vi "Default.vi"(8 "error in (no error)":errorcluster, 11 "CallEXEStep in":refnum<class "CallEXEStep.lvclass">) -> (0 "error out":errorcluster, 3 "CallEXEStep out":refnum<class "CallEXEStep.lvclass">)   [LabVIEW 2015, in "CallEXEStep.lvclass"]
uses:
  CallEXEStep.lvclass
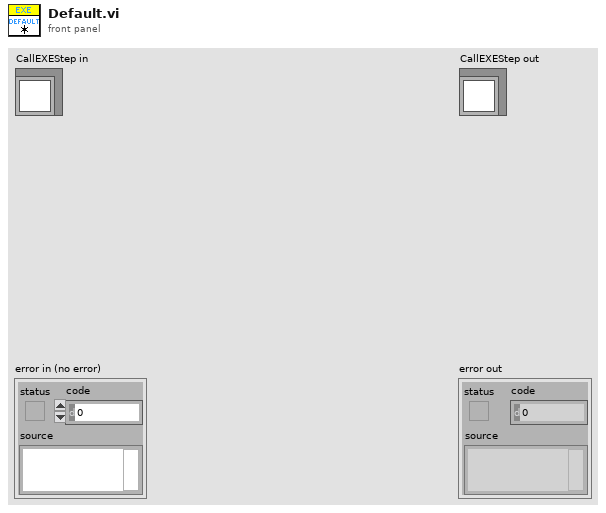
[diagram p1: front panel]
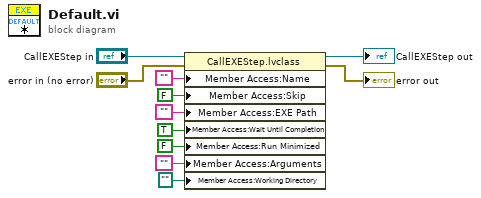
[diagram p0: block diagram]
diagram:
  n1 = property class="CallEXEStep.lvclass"(reference="CallEXEStep in", error in="error in (no error)", "Member Access:Name"="", "Member Access:Skip"=FALSE ("Skip"), "Member Access:EXE Path"="", "Member Access:Wait Until Completion"=TRUE ("Skip"), "Member Access:Run Minimized"=FALSE ("Run Minimized"), "Member Access:Arguments"="", "Member Access:Working Directory"=path "") -> (reference out=→"CallEXEStep out":refnum<class "CallEXEStep.lvclass">, error out=→"error out":errorcluster)
